vi "Replace File.vi"(1 "File In":path) -> (0 "File Out":path)   [LabVIEW 2017, in "DocTools.lvlib"]
uses:
  DocTools.lvlib
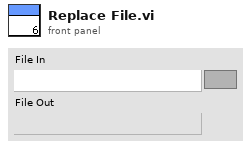
[diagram p1: front panel]
types:
  T1 = enum16{"open", "replace", "create", "open or create", "replace or create", "replace or create with confirmation"}
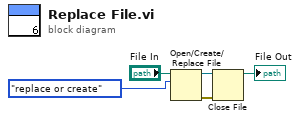
[diagram p0: block diagram]
diagram:
  n1 = Open/Create/Replace File(file path (use dialog)="File In", operation (0:open)=T1."replace or create") -> (refnum out=w2:refnum<file>, error out=w5:errorcluster)  [unwired: 4 in, 1 out]
  n2 = Close File(refnum=w2, error in=w5) -> (path=→"File Out":path)  [unwired: 1 out]
